vi "Set Point.vi"(8 "error in (no error)":errorcluster, 9 "Output #":i32=1, 10 "Set point":dbl, 11 "Temperature Controller in":refnum<class "Temperature Controller.lvclass">) -> (0 "error out":errorcluster, 3 "Temperature Controller out":refnum<class "Temperature Controller.lvclass">)   [LabVIEW 2021, in "Temperature Controller.lvclass"]
uses:
  Temperature Controller.lvclass
  Read T ctl driver.vi
  Write T ctl driver.vi
  NHMFL_Core/Libraries/Instruments/Temperature Controller Driver/Temperature Controller Driver.lvclass
  Temperature Controller.lvclass/Temperature Controller.ctl
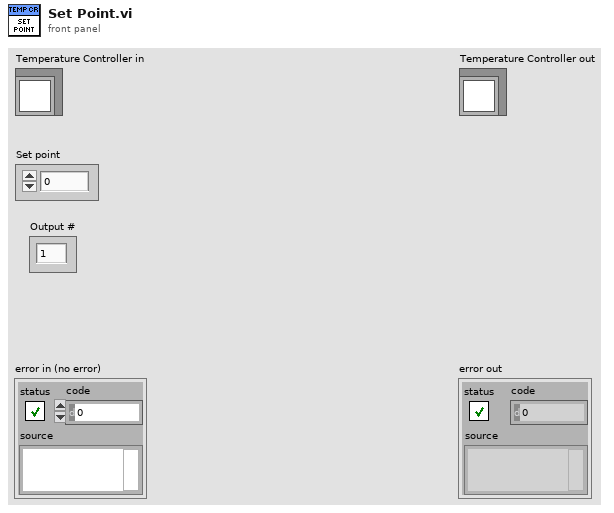
[diagram p1: front panel]
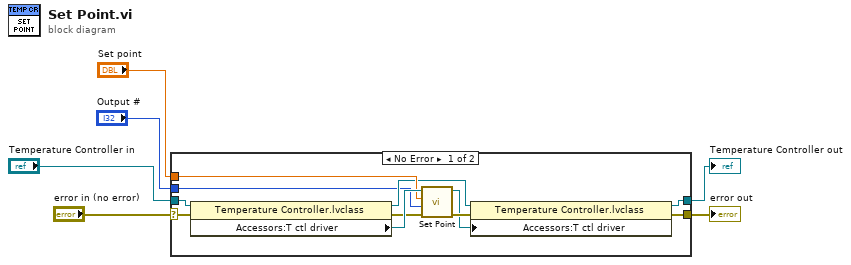
[diagram p0: block diagram]
diagram:
  n1 = case shown="No Error" "error in (no error)" {
    selector: "error in (no error)" -> [w17 w19]
    tunnel: [w13 w19] -> w5
    tunnel: [w11 w18] -> w3
    tunnel: "Temperature Controller in" -> [w16 w18]
    tunnel: "Set point" -> [w14 _]
    tunnel: "Output #" -> [w7 _]
    frame No Error {
      n2 = property class="Temperature Controller.lvclass"(reference=w16, error in=w17) -> (reference out=w12:refnum<class "Temperature Controller.lvclass">, error out=w10:errorcluster, "Accessors:T ctl driver"=w15:refnum<class "Temperature Controller Driver.lvclass">)
      n3 = call-dynamic "Set Point.vi"("error in (no error)"=w10, "Output #"=w7, "Set point"=w14, "Temperature Controller Driver in"=w15) -> ("error out"=w9:errorcluster, "Temperature Controller Driver out"=w8:refnum<class "Temperature Controller Driver.lvclass">)  [unwired: 6 in]
      n4 = property class="Temperature Controller.lvclass"(reference=w12, error in=w9, "Accessors:T ctl driver"=w8) -> (reference out=w11:refnum<class "Temperature Controller.lvclass">, error out=w13:errorcluster)
    }
    frame Error {
    }
  }
  "error out" <- w5
  "Temperature Controller out" <- w3
